vi "testSubEventCpp.vi"(8 "error in (no error)":errorcluster) -> (0 "error out":errorcluster)   [LabVIEW 2018]
uses:
  src/SalProcess/SalProcess.lvclass
  <vilib>/addons/_JKI Toolkits/Caraya/classes/Assert/Assert Equal Value_Variant.vi
  <vilib>/addons/_JKI Toolkits/Caraya/classes/Test/Test.lvclass
  <vilib>/addons/_JKI Toolkits/Caraya/classes/Assert/Assert.lvclass
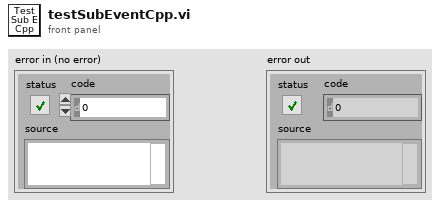
[diagram p1: front panel]
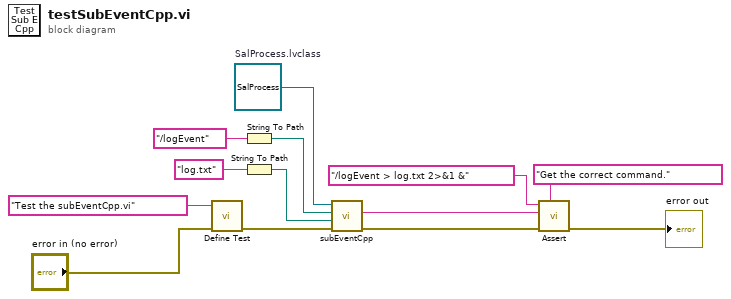
[diagram p0: block diagram]
diagram:
  w13 = refnum<class "SalProcess.lvclass"> refnum  # SalProcess.lvclass
  n1 = call <vilib>:"Define Test.vi"("error in (no error)"="error in (no error)", "Label (VI Title)"="Test the subEventCpp.vi") -> ("error out"=w10:errorcluster)  [unwired: 9 in]
  n2 = String To Path(string="/logEvent") -> (path=w8:path)
  n3 = String To Path(string="log.txt") -> (path=w6:path)
  n4 = call "subEventCpp.vi"("error in (no error)"=w10, "pathOfOutput"=w6, "pathOfSubEvent"=w8, "SalProcess in"=w13) -> ("error out"=w5:errorcluster, "cmd"=w4:string)  [unwired: 5 in, 1 out]
  n5 = call-poly <vilib>:"Assert.vi"("Label"="Get the correct command.", "error in (no error)"=w5, "Y"=w4, "X"="/logEvent > log.txt 2>&1 &" ("Display")) -> ("error out"=→"error out":errorcluster)  [unwired: 7 in]
